vi "command_move_absolute.vi"(8 "error in (no error)":errorcluster, 10 "target  position":refnum<class "SpaceVector.lvclass">, 11 "StageMH110930Scientifica in":refnum<class "StageMMS2015ASIfromScientifica.lvclass">) -> (0 "error out":errorcluster, 3 "StageMH110930Scientifica out":refnum<class "StageMMS2015ASIfromScientifica.lvclass">)   [LabVIEW 2010, in "StageMMS2015ASIfromScientifica.lvclass"]
uses:
  StageMMS2015ASIfromScientifica.lvclass
  common/classes/SpaceVector/SpaceVector/SpaceVector.lvclass
  common/classes/ErrorController/ErrorController/class_data.vi
  common/classes/ErrorController/ErrorController/ErrorController.lvclass
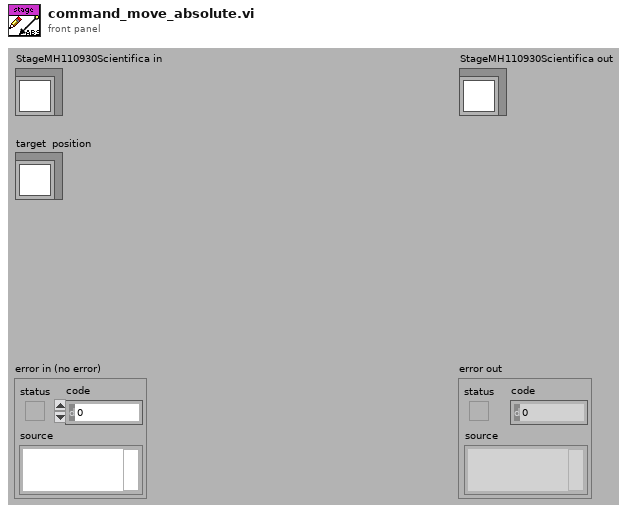
[diagram p1: front panel]
types:
  T1 = typedef "SpaceVector.lvclass/space_vector_array.ctl" = dbl[unit][]
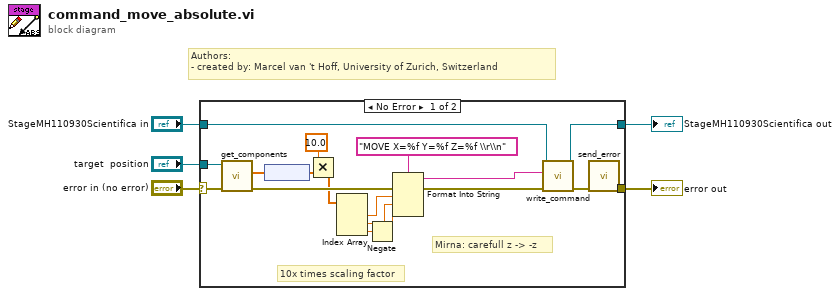
[diagram p0: block diagram]
diagram:
  # "Authors: \n- created by: Marcel van 't Hoff, University of Zurich, Switzerland"
  n1 = case shown="No Error" "error in (no error)" {
    selector: "error in (no error)" -> [w22 w25]
    tunnel: [w12 w25] -> w4
    tunnel: [w13 w24] -> w2
    tunnel: "StageMH110930Scientifica in" -> [w14 w24]
    tunnel: "target  position" -> [w23 _]
    frame No Error {
      # "Mirna: carefull z -> -z"
      # "10x times scaling factor"
      n2 = call "get_components.vi"("error in (no error)"=w22, "SpaceVector in"=w23) -> ("error out"=w16:errorcluster, "x/y/z"=w21:T1)  [unwired: 8 out]
      n3 = node(w21) -> (w11:dbl[])
      n4 = Multiply(x=10.0, y=w11) -> (x*y=w9:dbl[])
      n5 = Index Array(array=w9) -> (element #1=w20:dbl, element #2=w19:dbl, element #3=w18:dbl)  [unwired: 3 in]
      n6 = Negate(x=w18) -> (-x=w7:dbl)
      n7 = Format Into String(format string="MOVE X=%f Y=%f Z=%f \\r\\n", error in=w16, w20, w19, w7) -> (resulting string=w17:string, error out=w15:errorcluster)  [unwired: 1 in]
      n8 = call-dynamic "write_command.vi"("error in (no error)"=w15, "string to write"=w17, "StageMH110930Scientifica in"=w14) -> ("error out"=w10:errorcluster, "StageMH110930Scientifica out"=w13:refnum<class "StageMMS2015ASIfromScientifica.lvclass">)  [unwired: 5 in, 2 out]
      n9 = call "send_error.vi"("error in (no error)"=w10) -> ("error out"=w12:errorcluster)  [unwired: 10 in]
    }
    frame Error {
    }
  }
  "error out" <- w4
  "StageMH110930Scientifica out" <- w2
